vi "Get Status.vi"(8 "error in (no error)":errorcluster, 11 "Reader.lvclass in":refnum<class "Reader.lvclass">) -> (0 "error out":errorcluster, 2 "Status":string, 3 "Reader.lvclass out":refnum<class "Reader.lvclass">)   [LabVIEW 2009, in "Reader.lvclass"]
uses:
  Reader.lvclass
  Instruments/Utility Classes/Readable/Readable.lvclass
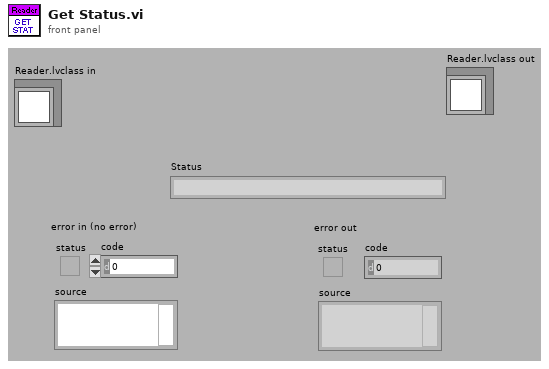
[diagram p1: front panel]
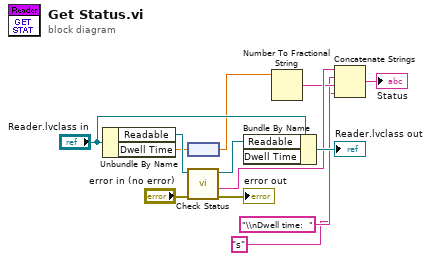
[diagram p0: block diagram]
diagram:
  n1 = Unbundle By Name("Reader.lvclass in") -> ("Readable"=w13:refnum<class "Readable.lvclass">, "Dwell Time"=w5:dbl[unit])
  n2 = node(w5) -> (w4:dbl)
  n3 = call-dynamic "Check Status.vi"("error in (no error)"="error in (no error)", "Instrument in"=w13) -> ("error out"=→"error out":errorcluster, "Status"=w7:string, "Instrument out"=w11:refnum<class "Readable.lvclass">)  [unwired: 6 in, 1 out]
  n4 = Bundle By Name(cluster="Reader.lvclass in", "Readable"=w11) -> (→"Reader.lvclass out":refnum<class "Reader.lvclass">)  [unwired: 1 in]
  n5 = Number To Fractional String(number=w4) -> (F-format string=w3:string)  [unwired: 3 in]
  n6 = Concatenate Strings(w7, "\\nDwell time:  ", w3, "s") -> (→"Status":string)
